vi "Start Module.vi"(6 "Show Main VI Diagram on Init (F)":bool, 8 "error in":errorcluster, 11 "Database Manager in":refnum<class "Database Manager.lvclass">) -> (0 "error out":errorcluster, 1 "Wait for Event Sync?":bool, 2 "Database Manager Broadcast Events":T1, 3 "Module Was Already Running?":bool, 4 "Module Name":string)   [LabVIEW 2021, in "Database Manager.lvlib"]
doc: "Launches the module Main VI. After calling this VI, you can optionally register for broadcast events from the module by wiring the broadcast events output of this VI to a <b>Register For Events</b> function. \n\nAfter the optional Register For Events function call, you should always call the <b>Synchronize Module Events.vi</b> for this module with the 'Wait for Event Sync?' output of this VI to the corresponding input of the Synchronize Module Events.vi. \n\nTo see an example of the proper wiring pattern, see the \"Start Module: Value Change\" event frame in the API Tester VI for this module.\n\nThe <b>Validate DQMH Module</b> tool added a 'Module Name' output to this VI.\n_____\nBased on DQMH Dev Tools: Project Template 7.1.2.1547."
uses:
  Database Manager.lvlib
  Broadcast Events--cluster.ctl
  Did Init Argument--cluster.ctl
  Status Updated Argument--cluster.ctl
  Error Reported Argument--cluster.ctl
  Stop Argument--cluster.ctl
  Get Module Execution Status Argument--cluster.ctl
  Database Manager/Database Manager.lvclass
  <vilib>/Delacor/Delacor QMH/Libraries/Module Admin_class/Delacor_lib_QMH_Module Admin.lvclass
  <vilib>/Delacor/Delacor QMH/Libraries/Module Admin_class/Delacor_lib_QMH_Module Admin.lvclass/Delacor_lib_QMH_Module Admin.ctl
  <vilib>/Delacor/Delacor QMH/Libraries/Module Admin_class/Delacor_lib_QMH_Set External Launch.vi
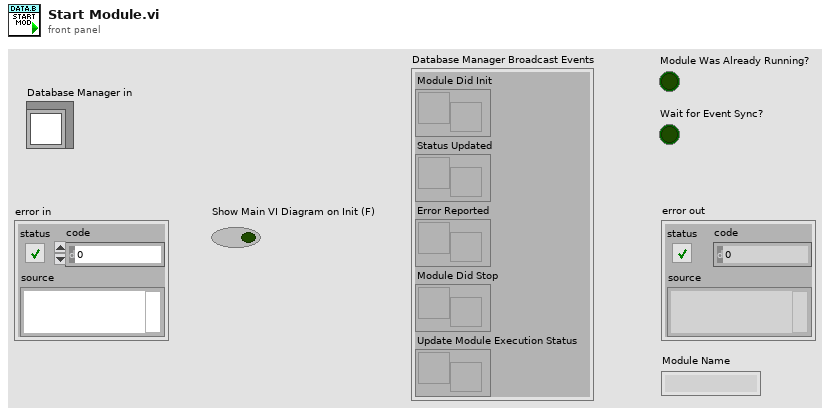
[diagram p1: front panel]
types:
  T1 = typedef "Database Manager.lvlib/Broadcast Events--cluster.ctl" = cluster{"Module Did Init":refnum<user-event>, "Status Updated":refnum<user-event>, "Error Reported":refnum<user-event>, "Module Did Stop":refnum<user-event>, "Update Module Execution Status":refnum<user-event>}
  T2 = enum32{"Bad", "Idle", "Run top level", "Running"}
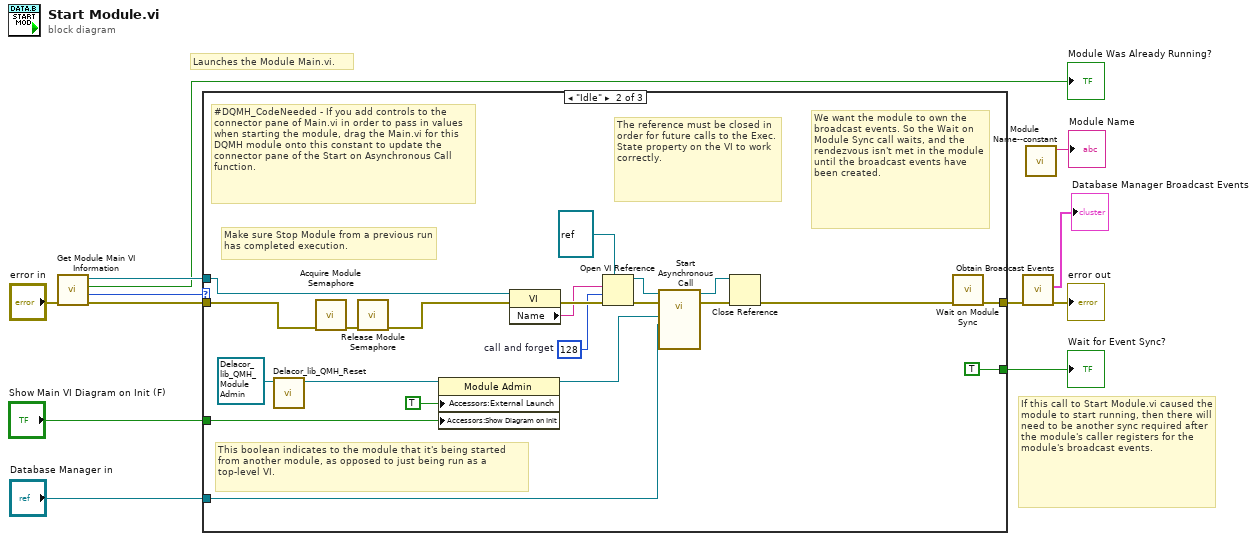
[diagram p0: block diagram]
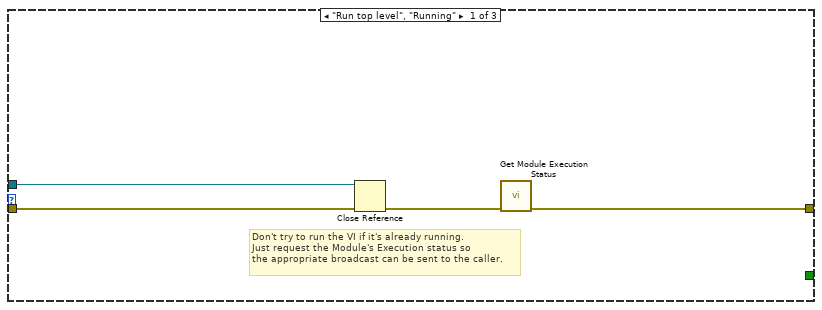
[diagram p2: hidden frame]
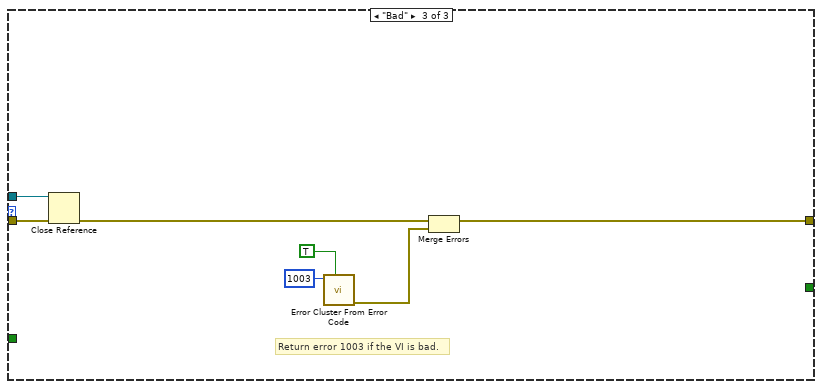
[diagram p3: hidden frame]
diagram:
  # "If this call to Start Module.vi caused the module to start running, then there will need to be another sync required after the module's caller registers for the module's broadcast events."
  # "Launches the Module Main.vi."
  n1 = call "Get Module Main VI Information.vi"("error in"="error in") -> ("error out"=w12:errorcluster, "Execution State"=w7:T2, "Is Module Running?"=→"Module Was Already Running?":bool, "Module Main VI"=w11:refnum<vi>)  [unwired: 7 in]
  n2 = case shown="\"Idle\"" w7 {
    tunnel: w12 -> [w16 w20 w44]
    tunnel: w11 -> [w15 w32 w43]
    tunnel: [w13 w37 w41] -> w10
    tunnel: [_ TRUE _] -> w8
    tunnel: "Show Main VI Diagram on Init (F)" -> [_ w18 _]
    tunnel: "Database Manager in" -> [_ w17 _]
    frame "Run top level", "Running" {
      # "Don't try to run the VI if it's already running.\nJust request the Module's Execution status so\nthe appropriate broadcast can be sent to the caller."
      n3 = Close Reference(reference=w15, error in (no error)=w16) -> (error out=w14:errorcluster)
      n4 = call "Get Module Execution Status.vi"("error in"=w14) -> ("error out"=w13:errorcluster)  [unwired: 10 in]
    }
    frame "Idle" {
      w29 = 128  # call and forget
      # "Make sure Stop Module from a previous run has completed execution."
      # "#DQMH_CodeNeeded - If you add controls to the connector pane of Main.vi in order to pass in values when starting the module, drag the Main.vi for this DQMH module onto this constant to update the connector pane of the Start on Asynchronous Call function."
      # "The reference must be closed in order for future calls to the Exec.State property on the VI to work correctly."
      # "We want the module to own the broadcast events. So the Wait on Module Sync call waits, and the rendezvous isn't met in the module until the broadcast events have been created."
      # "This boolean indicates to the module that it's being started from another module, as opposed to just being run as a top-level VI."
      n5 = call-dynamic "Delacor_lib_QMH_Reset.vi"("Mod Admin in"=refnum<class "Delacor_lib_QMH_Module Admin.lvclass"> refnum) -> ("Mod Admin out"=w35:refnum<class "Delacor_lib_QMH_Module Admin.lvclass">)  [unwired: 9 in, 1 out]
      n6 = call "Acquire Module Semaphore.vi"("error in"=w20) -> ("error out"=w21:errorcluster)  [unwired: 10 in]
      n7 = call "Release Module Semaphore.vi"("error in"=w21) -> ("error out"=w19:errorcluster)  [unwired: 10 in]
      n8 = property class="Module Admin"(reference=w35, "Accessors:External Launch"=TRUE, "Accessors:Show Diagram on Init"=w18) -> (reference out=w26:refnum<class "Delacor_lib_QMH_Module Admin.lvclass">)  [unwired: 1 in, 1 out]
      n9 = property class="VI"(reference=w32, error in=w19) -> (error out=w31:errorcluster, "Name"=w22:string)  [unwired: 1 out]
      n10 = Open VI Reference(type specifier VI Refnum (for type only)=refnum<vi> refnum, vi path=w22, options=w29, error in (no error)=w31) -> (vi reference=w27:refnum<vi>, error out=w28:errorcluster)  [unwired: 2 in]
      n11 = call-by-ref "Start Asynchronous Call"(reference=w27, error in=w28, "Database Manager in"=w17, "Module Admin"=w26) -> (reference out=w24:refnum<vi>, error out=w25:errorcluster)  [unwired: 10 in]
      n12 = Close Reference(reference=w24, error in (no error)=w25) -> (error out=w23:errorcluster)
      n13 = call "Wait on Module Sync.vi"("error in"=w23) -> ("error out"=w37:errorcluster)  [unwired: 10 in]
    }
    frame "Bad" {
      # "Return error 1003 if the VI is bad."
      n14 = Close Reference(reference=w43, error in (no error)=w44) -> (error out=w42:errorcluster)
      n15 = call <vilib>:"Error Cluster From Error Code.vi"("show call chain? (False)"=TRUE, "error code (0)"=1003) -> ("error out"=w40:errorcluster)  [unwired: 7 in]
      n16 = Merge Errors(w42, w40) -> (w41:errorcluster)
    }
  }
  "Wait for Event Sync?" <- w8
  n17 = call "Obtain Broadcast Events.vi"("error in"=w10) -> ("error out"=→"error out":errorcluster, "Database Manager Broadcast Events"=→"Database Manager Broadcast Events":T1)  [unwired: 9 in]
  n18 = call "Module Name--constant.vi"() -> ("Module Name"=→"Module Name":string)  [unwired: 11 in]
